vi "GUI_Sam_temp.vi"() -> ()   [LabVIEW 2013]
uses:
  shared programs/GUI_Template/GUI_master/tcp_new_data_event.ctl
  shared programs/GUI_Template/GUI_master/tcp new data cluster.ctl
panel:
  out "image::7":T1(plugin-control) caption="U_Amp3GaiaBay"
  in  "triggerdelay::7":dbl=0.001 caption="triggerdelay" min=0.0 max=50000.0 format="%_4p"
  in  "triggerdelay::6":dbl=0.001 caption="triggerdelay" min=20.0 max=50000.0 format="%_4p"
  in  "triggerdelay::5":dbl=0.001 caption="triggerdelay" min=10.0 max=50000.0 format="%_4p"
  in  "triggerdelay::4":dbl=0.001 caption="triggerdelay" min=0.0 max=50000.0 format="%_4p"
  in  "triggerdelay::3":dbl=0.001 caption="triggerdelay" min=20.0 max=50000.0 format="%_4p"
  in  "triggerdelay::2":dbl=0.001 caption="triggerdelay" min=0.0 max=50000.0 format="%_4p"
  in  "trigger::7":bool caption="Trigger"
  in  "centroidy::7":dbl=0.001 caption="centroid y" min=0.0 max=0.0 format="%_4f"
  in  "centroidx::7":dbl=0.001 caption="centroid x" min=0.0 max=0.0 format="%_4f"
  in  "exposure::7":dbl=0.001 caption="exposure" min=0.0001 max=1.0 format="%_4p"
  in  "GUIdevice 7":string="U_GAIACam"
  in  "trigger::6":bool caption="Trigger"
  in  "centroidy::6":dbl=0.001 caption="centroid y" min=0.0 max=0.0 format="%_4f"
  in  "centroidx::6":dbl=0.001 caption="centroid x" min=0.0 max=0.0 format="%_4f"
  in  "exposure::6":dbl=0.001 caption="exposure" min=0.0001 max=1.0 format="%_4p"
  out "image::6":T1(plugin-control) caption="U_Amp3GaiaBay"
  in  "GUIdevice 6":string="U_Amp3GaiaBay"
  in  "trigger::5":bool caption="Trigger"
  in  "centroidy::5":dbl=0.001 caption="centroid y" min=0.0 max=0.0 format="%_4f"
  in  "centroidx::5":dbl=0.001 caption="centroid x" min=0.0 max=0.0 format="%_4f"
  in  "exposure::5":dbl=0.001 caption="exposure" min=0.0001 max=1.0 format="%_4p"
  out "image::5":T1(plugin-control) caption="U_Amp2GaiaBay"
  in  "GUIdevice 5":string="U_Amp2GaiaBay"
  in  "trigger::4":bool caption="Trigger"
  in  "centroidy::4":dbl=0.001 caption="centroid y" min=0.0 max=0.0 format="%_4f"
  in  "centroidx::4":dbl=0.001 caption="centroid x" min=0.0 max=0.0 format="%_4f"
  in  "exposure::4":dbl=0.001 caption="exposure" min=1e-06 max=1.0 format="%_4p"
  out "image::4":T1(plugin-control) caption="U_IRMobileImager"
  in  "GUIdevice 4":string="U_IRMobileImager"
  in  "trigger::3":bool caption="Trigger"
  in  "centroidy::3":dbl=0.001 caption="centroid y" min=0.0 max=0.0 format="%_4f"
  in  "centroidx::3":dbl=0.001 caption="centroid x" min=0.0 max=0.0 format="%_4f"
  in  "exposure::3":dbl=0.001 caption="exposure" min=0.0001 max=1.0 format="%_4p"
  out "image::3":T1(plugin-control) caption="Amp3_IR_Input"
  in  "GUIdevice 3":string="U_Amp3_IR_Input"
  in  "trigger::2":bool caption="Trigger"
  in  "centroidy::2":dbl=0.001 caption="centroid y" min=0.0 max=0.0 format="%_4f"
  in  "centroidx::2":dbl=0.001 caption="centroid x" min=0.0 max=0.0 format="%_4f"
  in  "exposure::2":dbl=0.001 caption="exposure" min=0.0001 max=1.0 format="%_4p"
  out "image::2":T1(plugin-control) caption="Amp2_IR_input"
  in  "GUIdevice 2":string="U_Amp2_IR_input"
  out "tcp data event":T2
  in  "Refresh Button":bool
  in  "Select device":string(combo)="FrogHPD"
  in  "stop":bool
  in  "GUIdevice 1":string="HPD_CCD"
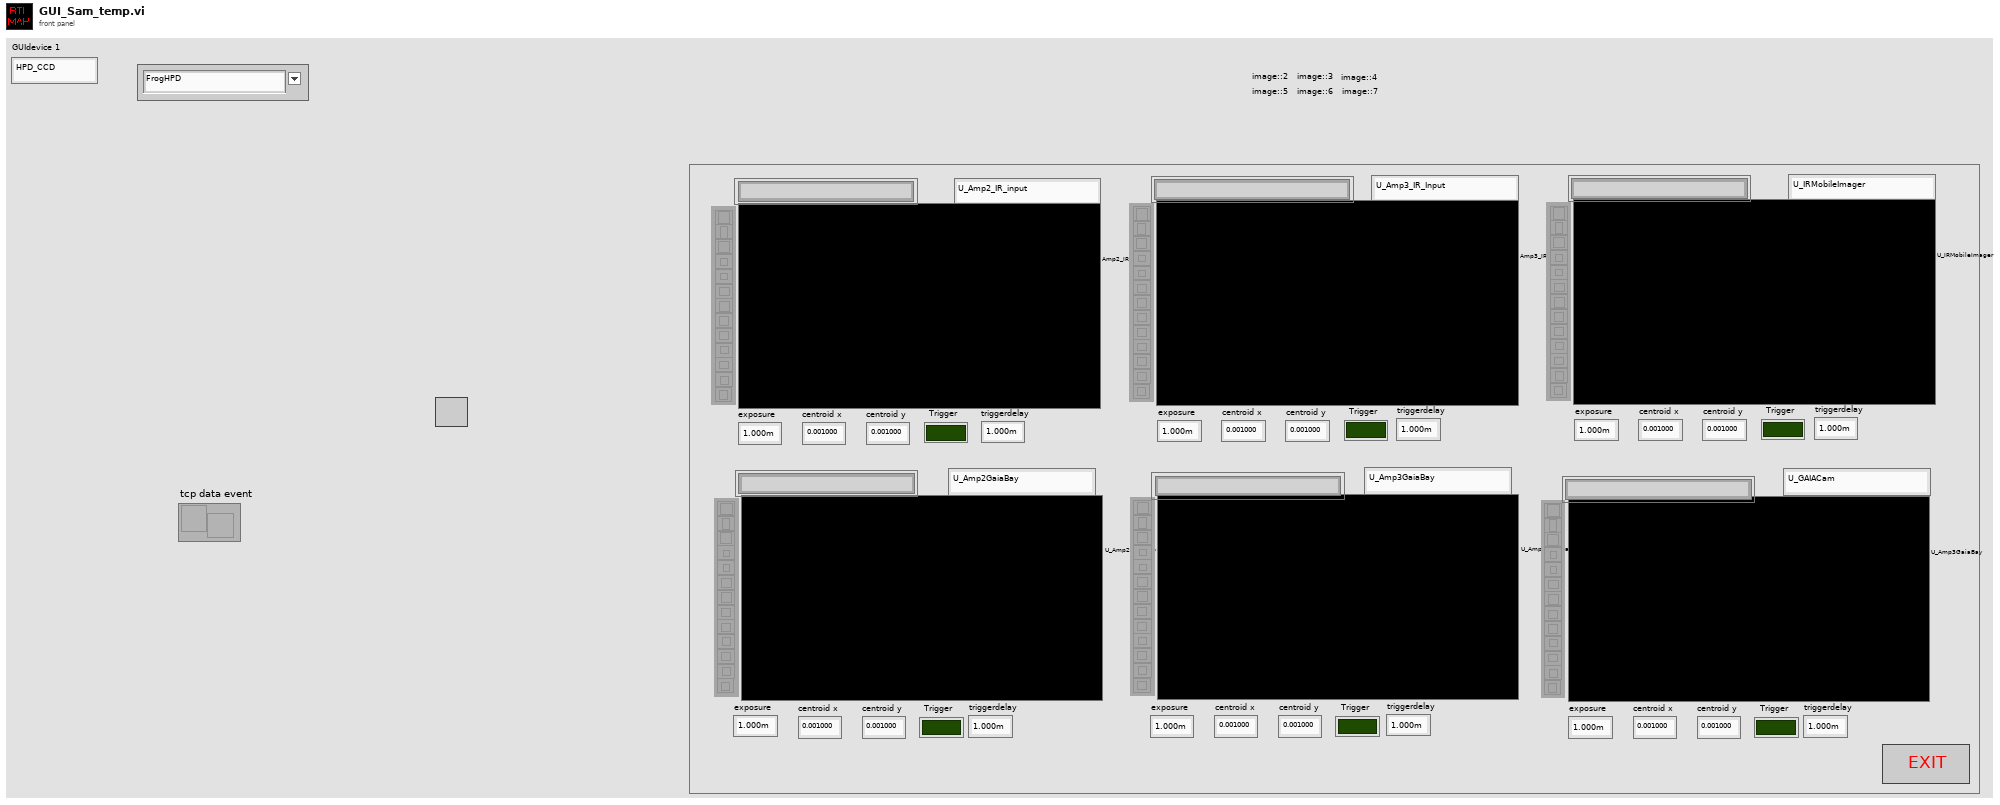
[diagram p1: front panel]
types:
  T1 = typedef "IMAQ Image.ctl" = refnum<image>
  T2 = typedef "tcp_new_data_event.ctl" = refnum<user-event>
  T3 = typedef "Image Type" = u32
  T4 = enum32{"invalid app kind", "Development System", "Run Time System", "Student Edition", "Embedded LabVIEW", "Evaluation", "Custom"}
  T5 = typedef "tcp new data cluster.ctl" = cluster{"EventEnum":enum16{"new data", "connection status update"}, "Device name":string}
  T6 = enum32{"Invalid", "Standard", "Closed", "Hidden", "Minimized", "Maximized"}
  T7 = cluster{"Core":cluster{"Current VI Reference":refnum<vi>, "Close Panel on Exit?":bool}, "Your Boolean data":bool, "Your string data":string, "SuperGUI":cluster{"STOP queue":refnum<queue>, "SuperGUI ref":refnum<vi>}}
  T8 = cluster{"STOP queue":refnum<queue>, "SuperGUI ref":refnum<vi>}
  T9 = cluster{"Current VI Reference":refnum<vi>, "Close Panel on Exit?":bool}
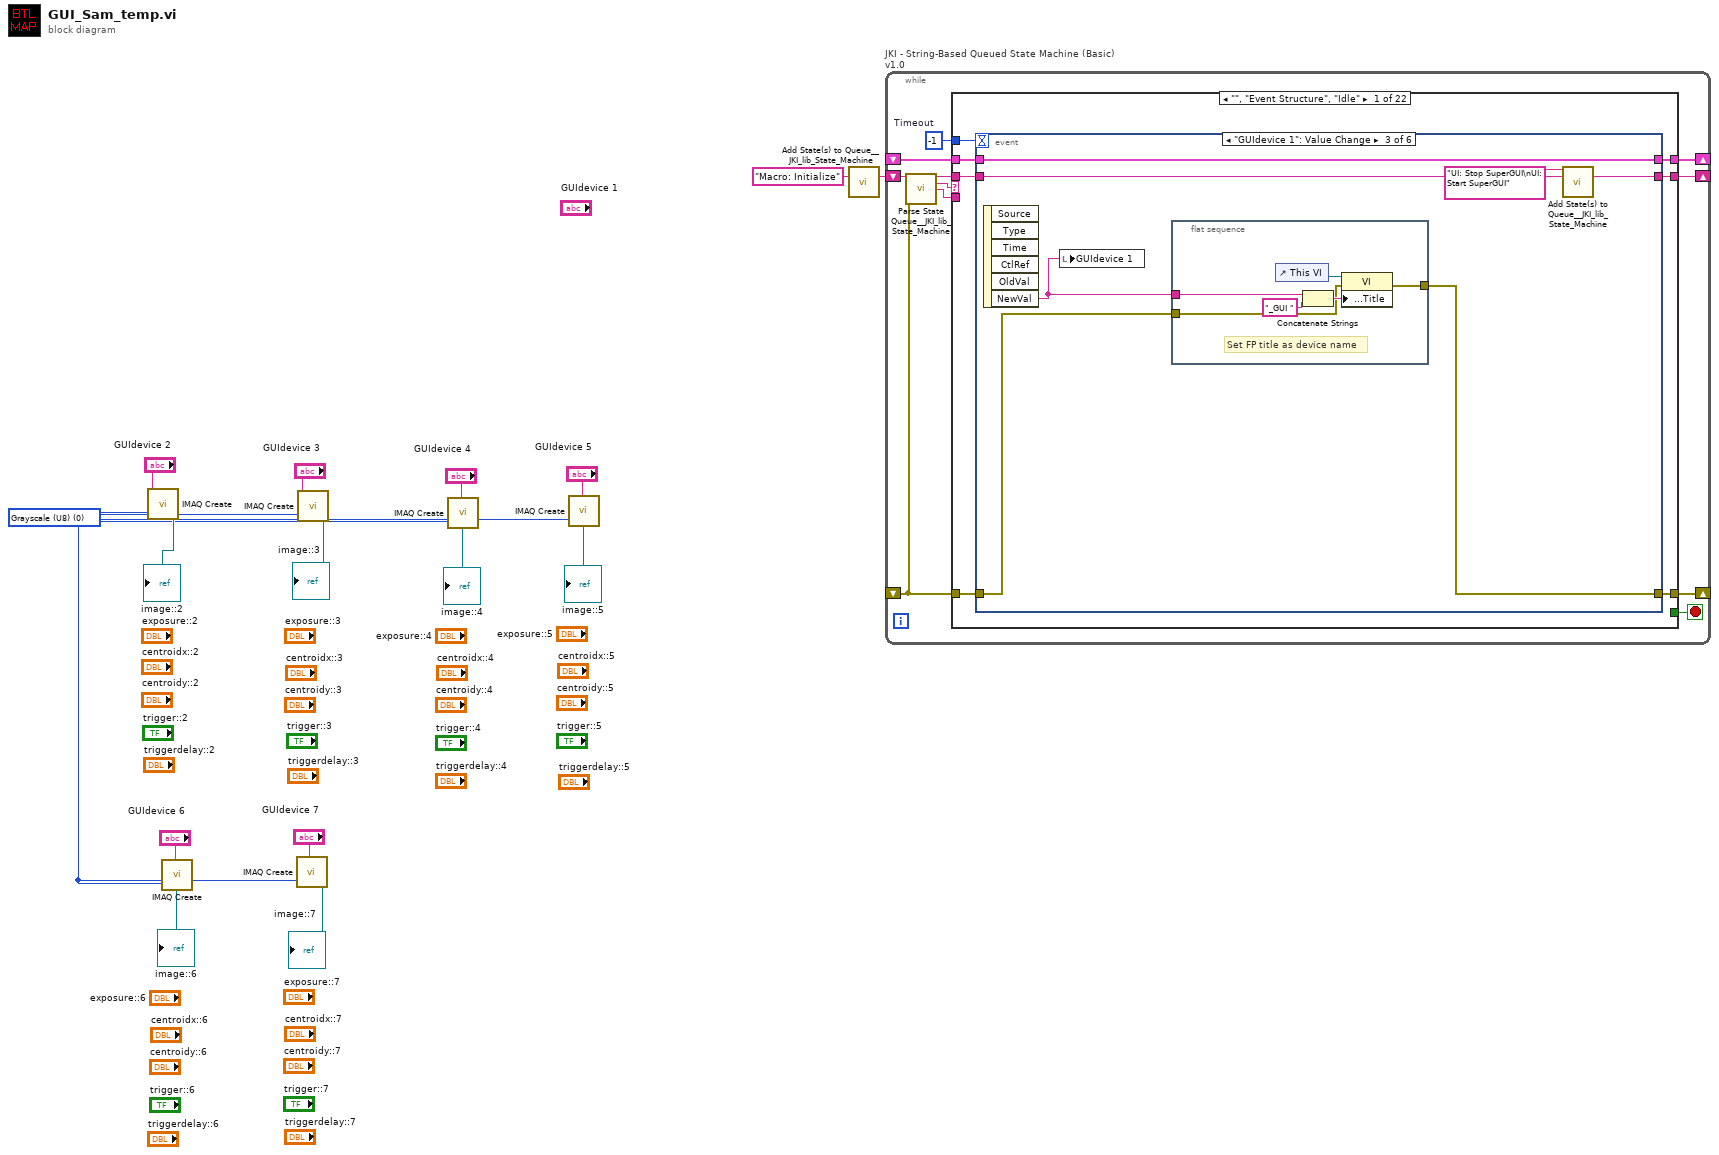
[diagram p0: block diagram]
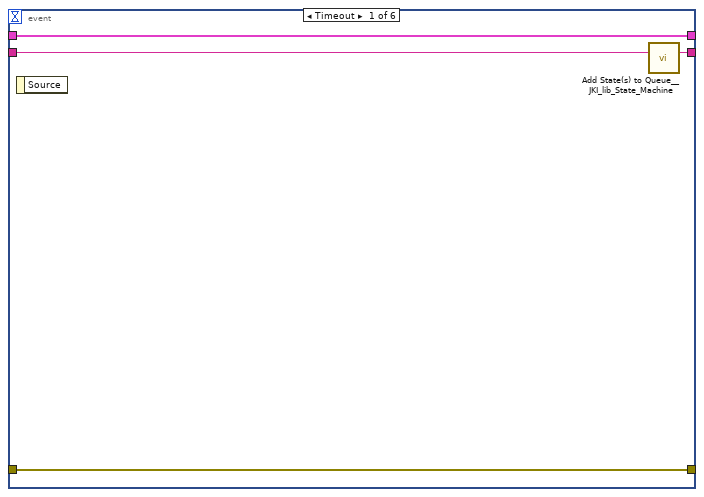
[diagram p2: hidden frame]
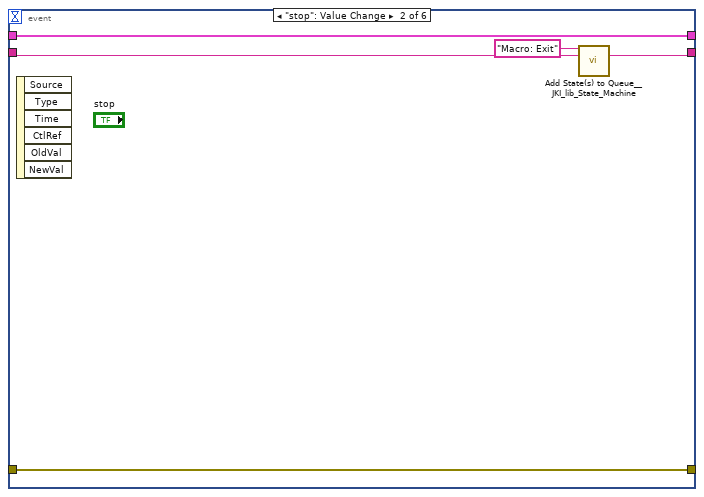
[diagram p3: hidden frame]
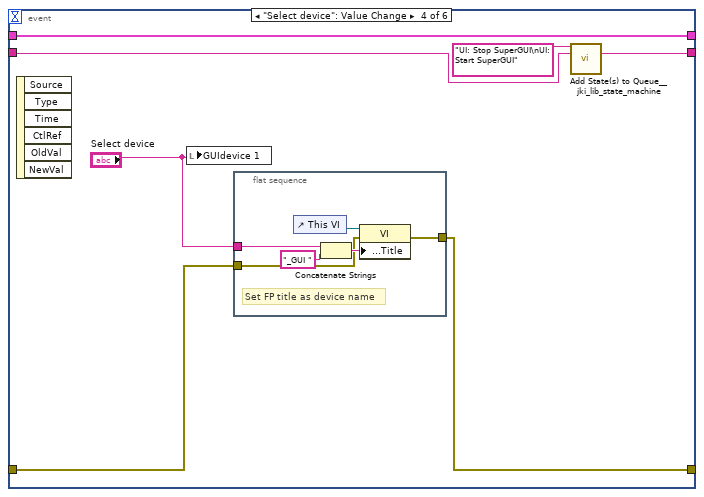
[diagram p4: hidden frame]
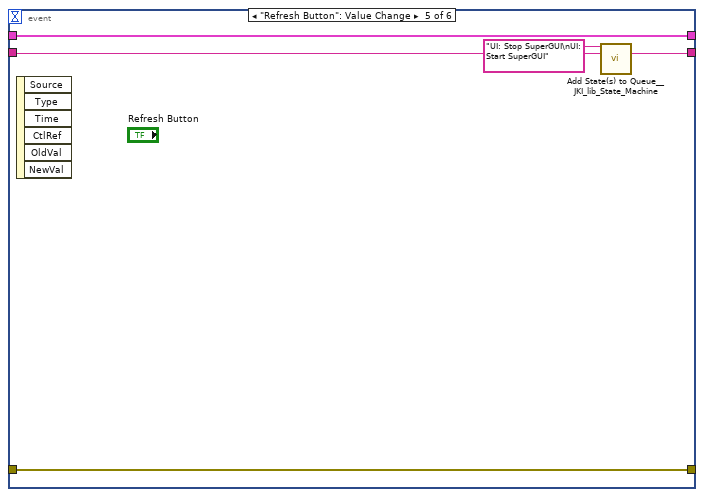
[diagram p5: hidden frame]
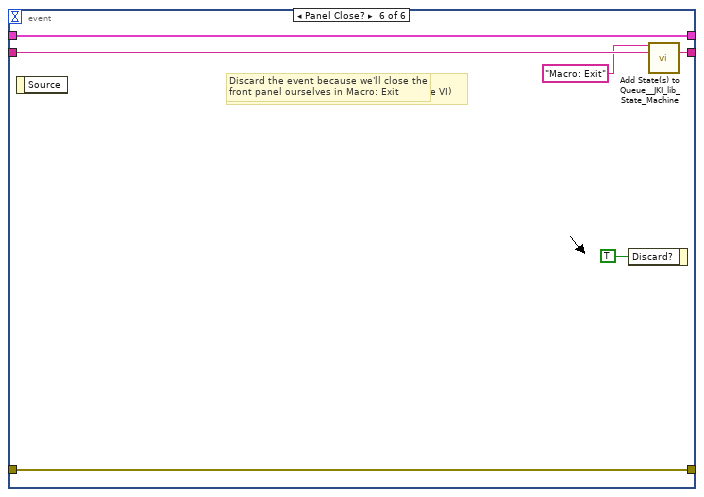
[diagram p6: hidden frame]
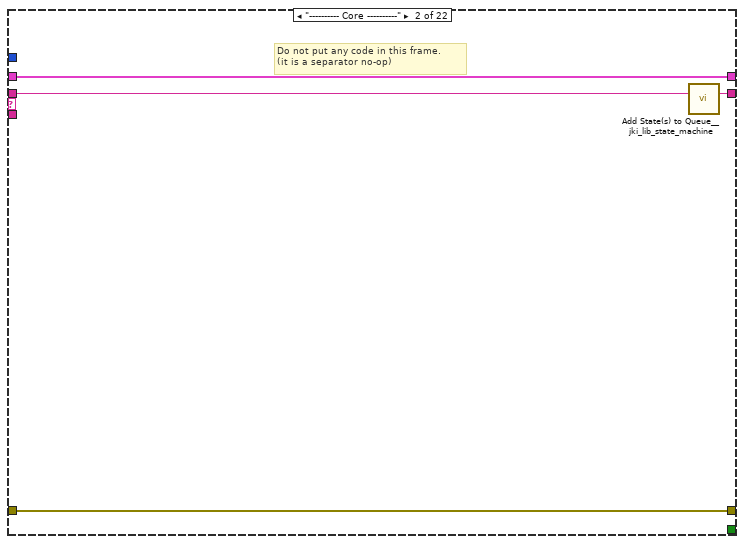
[diagram p7: hidden frame]
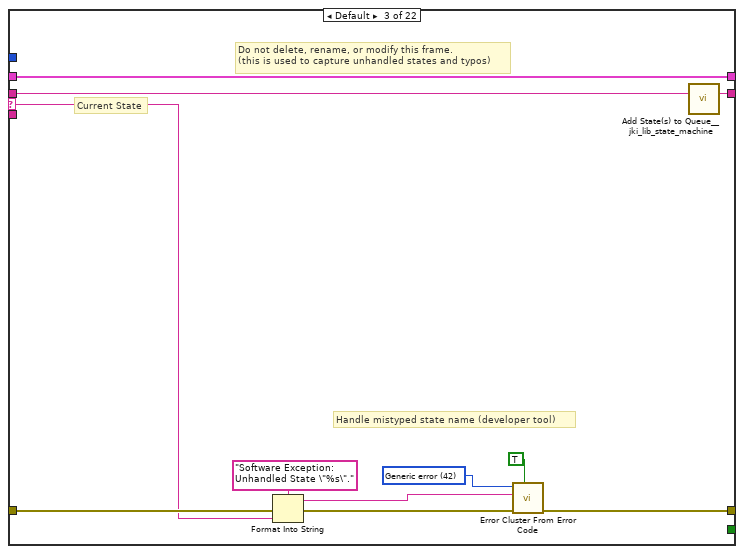
[diagram p8: hidden frame]
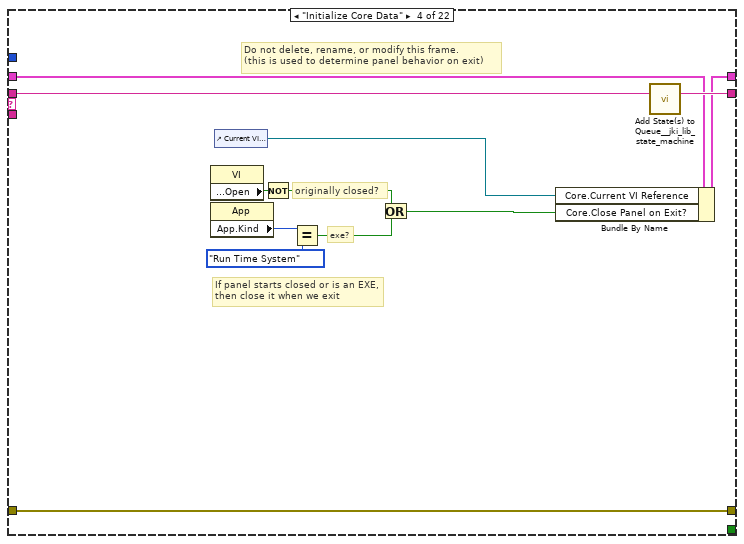
[diagram p9: hidden frame]
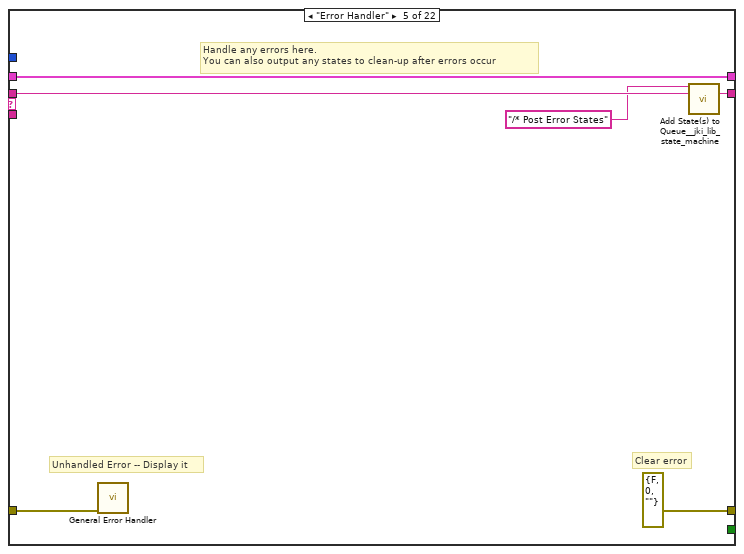
[diagram p10: hidden frame]
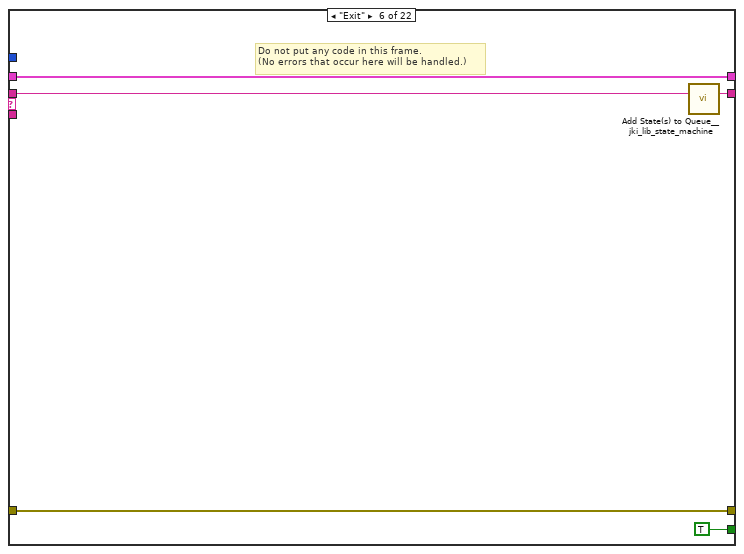
[diagram p11: hidden frame]
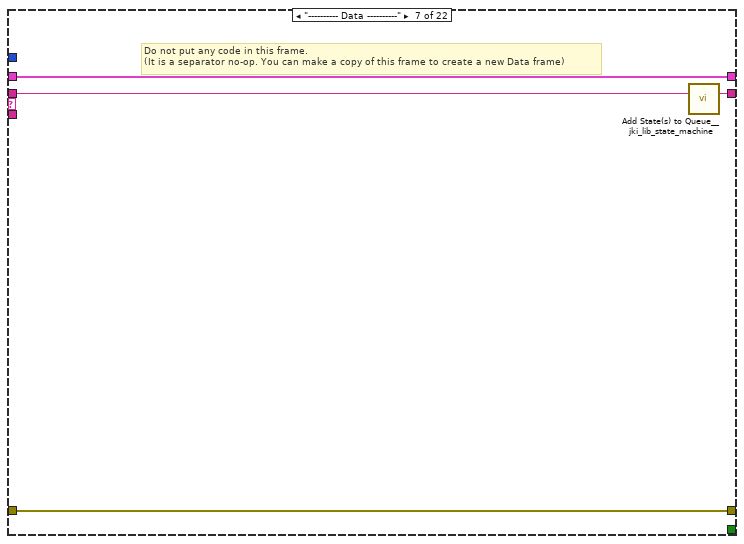
[diagram p12: hidden frame]
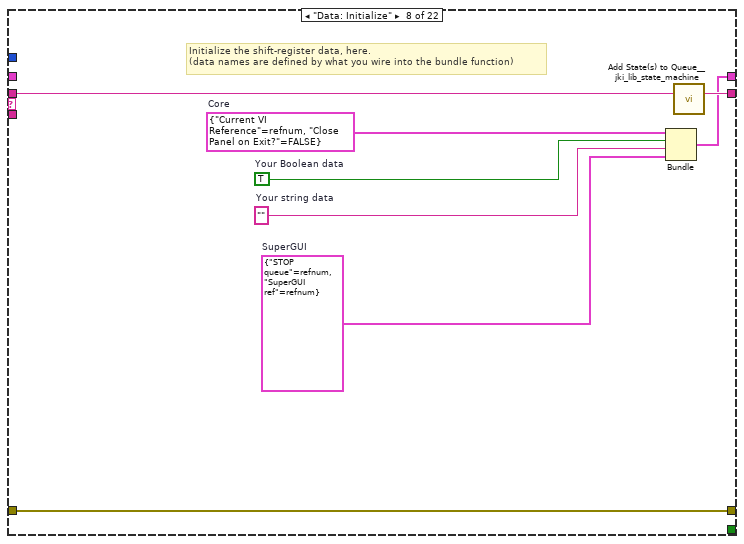
[diagram p13: hidden frame]
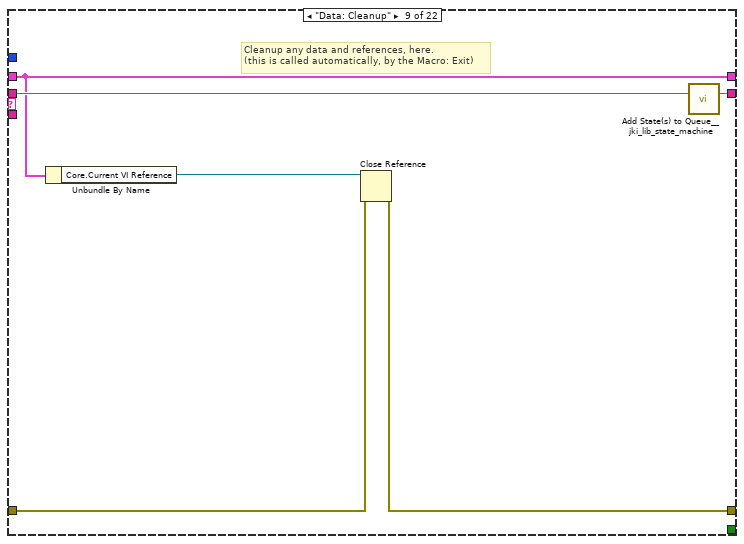
[diagram p14: hidden frame]
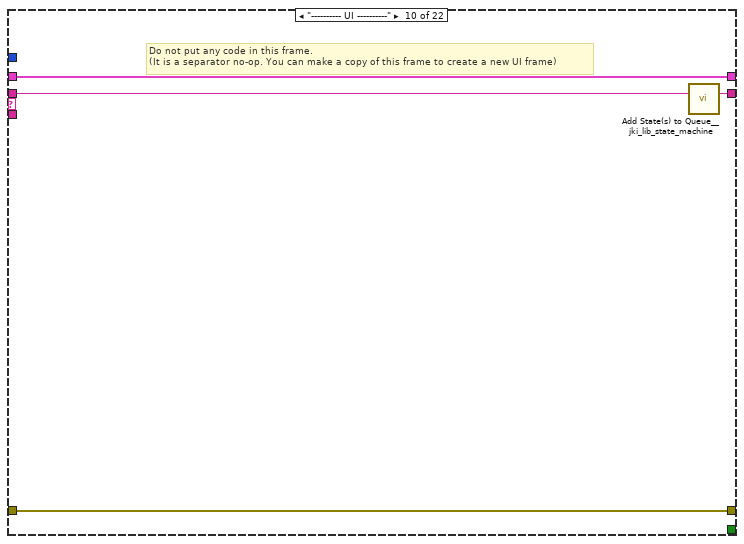
[diagram p15: hidden frame]
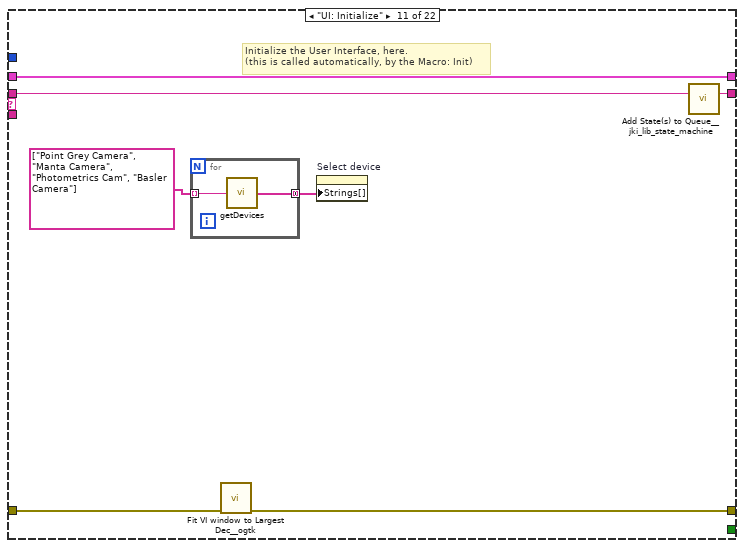
[diagram p16: hidden frame]
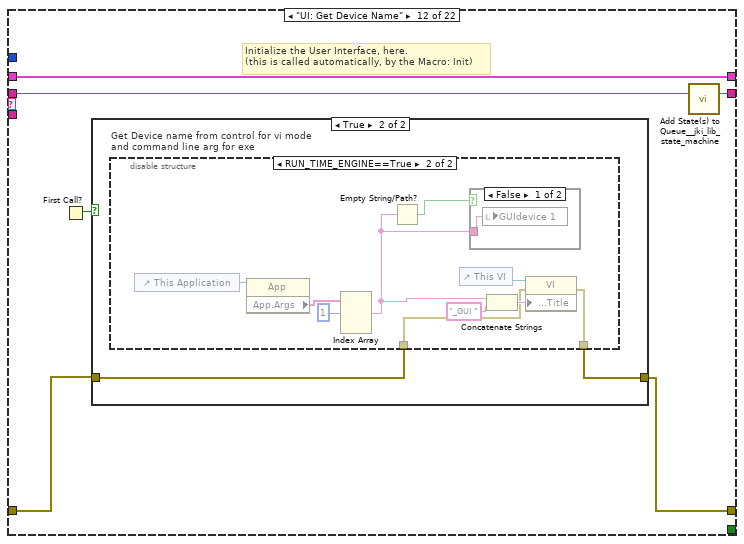
[diagram p17: hidden frame]
diagram:
  w2 = T3 0 items=["Grayscale (U8)", "Grayscale (I16)", "Grayscale (SGL)", "Complex (CSG)", "RGB (U32)", "HSL (U32)", "RGB (U64)", "Grayscale (U16)"] ("Image Type")
  n1 = call "IMAQ Create"("Image Name"="GUIdevice 2", "Image Type"=w2) -> ("New Image"=→"image::2":T1)  [unwired: 3 in, 1 out]
  n2 = call "IMAQ Create"("Image Name"="GUIdevice 6", "Image Type"=w2) -> ("New Image"=→"image::6":T1)  [unwired: 3 in, 1 out]
  n3 = call "IMAQ Create"("Image Name"="GUIdevice 7", "Image Type"=w2) -> ("New Image"=→"image::7":T1)  [unwired: 3 in, 1 out]
  n4 = call "IMAQ Create"("Image Name"="GUIdevice 3", "Image Type"=w2) -> ("New Image"=→"image::3":T1)  [unwired: 3 in, 1 out]
  n5 = call "IMAQ Create"("Image Name"="GUIdevice 4", "Image Type"=w2) -> ("New Image"=→"image::4":T1)  [unwired: 3 in, 1 out]
  n6 = call "IMAQ Create"("Image Name"="GUIdevice 5", "Image Type"=w2) -> ("New Image"=→"image::5":T1)  [unwired: 3 in, 1 out]
  n7 = call <vilib>:"Add State(s) to Queue__JKI_lib_State_Machine.vi"("State(s) in (\"\")"="Macro: Initialize") -> ("States Out"=w15:string)  [unwired: 14 in]
  n8 = while "JKI - String-Based Queued State Machine (Basic) v1.0" {
    shift-right: [w19] -> _
    shift-left: _ -> [w18]
    shift-right: [w22] -> _
    shift-left: _ -> [w16]
    shift-right: [w21] -> _
    shift-left: w15 -> [w23]
    stop <- w20 stop-if-true
    w17 = -1  # Timeout
    n9 = call <vilib>:"Parse State Queue__JKI_lib_State_Machine.vi"("State Queue"=w23, "Error In (no error)"=w16) -> ("Remaining States"=w25:string, "Current State"=w26:string, "Arguments"=w24:string)  [unwired: 11 in]
    n10 = case shown="\"\", \"Event Structure\", \"Idle\"" w26 {
      selector: w26 -> [_ _ w84 _ _ _ _ _ _ _ _ _ _ _ _ _ _ _ _ _ _ _]
      tunnel: w25 -> [w33 w83 w88 w106 w112 w117 w121 w129 w135 w139 w146 w154 w189 w197 w203 w214 w240 w245 w255 w259 w263 w267]
      tunnel: w24 -> [_ _ _ _ _ _ _ _ _ _ _ _ _ _ w198 w208 _ _ _ _ _ _]
      tunnel: w18 -> [w31 w80 w86 w97 w109 w115 w118 _ w130 w136 w144 w152 w180 w192 w201 w210 w237 w242 w252 w256 w260 w264]
      tunnel: [w30 w81 w90 w103 errorcluster {"status"=FALSE, "code"=0, "source"=""} ("error out") w114 w119 w126 w131 w137 w142 w149 w173 w190 w199 w211 w238 w243 w253 w257 w261 w265] -> w22
      tunnel: w16 -> [w29 w81 w89 w103 w108 w114 w119 w126 w132 w137 w143 w150 w174 w191 w200 w212 w238 w243 w253 w257 w261 w265]
      tunnel: [w32 w82 w87 w105 w111 w116 w120 w128 w134 w138 w145 w153 w188 w196 w202 w213 w239 w244 w254 w258 w262 w266] -> w21
      tunnel: [_ _ _ _ _ TRUE _ _ _ _ _ _ _ _ _ _ _ _ _ _ _ _] -> w20
      tunnel: [w28 w80 w86 w104 w109 w115 w118 w127 w130 w136 w144 w152 w179 w192 w201 w210 w237 w242 w252 w256 w260 w264] -> w19
      tunnel: w17 -> [w27 _ _ _ _ _ _ _ _ _ _ _ _ _ _ _ _ _ _ _ _ _]
      frame "", "Event Structure", "Idle" {
        n11 = event shown="[2] \"GUIdevice 1\": Value Change" {
          selector: _ -> [_ _ _ _ _ _]
          dyn-events: _ -> [_ _ _ _ _ _]
          timeout: w27 -> [_ _ _ _ _ _]
          tunnel: w33 -> [w37 w40 w46 w58 w71 w79]
          tunnel: [w36 w39 w45 w57 w70 w78] -> w32
          tunnel: w31 -> [w34 w42 w49 w62 w73 w76]
          tunnel: [w35 w41 w47 w60 w72 w77] -> w30
          tunnel: w29 -> [w35 w41 w48 w61 w72 w77]
          tunnel: [w34 w42 w49 w62 w73 w76] -> w28
          event Timeout {
            n12 = event-data() -> ()  [unwired: 1 in, 1 out]
            n13 = call <vilib>:"Add State(s) to Queue__JKI_lib_State_Machine.vi"("State(s) in (\"\")"=w37) -> ("States Out"=w36:string)  [unwired: 14 in]
          }
          event "stop": Value Change {
            n14 = event-data() -> ()  [unwired: 1 in, 6 out]
            n15 = call <vilib>:"Add State(s) to Queue__JKI_lib_State_Machine.vi"("State(s) in Front (\"\")"="Macro: Exit", "State(s) in (\"\")"=w40) -> ("States Out"=w39:string)  [unwired: 13 in]
          }
          event "GUIdevice 1": Value Change {
            n16 = event-data() -> ("NewVal"=w43:string)  [unwired: 1 in, 5 out]
            n17 = local write "GUIdevice 1"(w43) -> ()
            n18 = flat-sequence {
              tunnel: [w52] -> w47
              tunnel: w48 -> [w51]
              tunnel: w43 -> [w50]
              frame #0 {
                # "Set FP title as device name"
                n19 = control-ref of="This VI"() -> (w55:refnum<vi>)
                n20 = Concatenate Strings(w50, "_GUI ") -> (w54:string)
                n21 = property class="VI"(reference=w55, error in=w51, "Front Panel.Title"=w54) -> (error out=w52:errorcluster)  [unwired: 1 out]
              }
            }
            n22 = call <vilib>:"Add State(s) to Queue__JKI_lib_State_Machine.vi"("State(s) in Front (\"\")"="UI: Stop SuperGUI\nUI: Start SuperGUI", "State(s) in (\"\")"=w46) -> ("States Out"=w45:string)  [unwired: 13 in]
          }
          event "Select device": Value Change {
            n23 = event-data() -> ()  [unwired: 1 in, 6 out]
            n24 = local write "GUIdevice 1"("Select device") -> ()
            n25 = flat-sequence {
              tunnel: [w65] -> w60
              tunnel: w61 -> [w64]
              tunnel: "Select device" -> [w63]
              frame #0 {
                # "Set FP title as device name"
                n26 = control-ref of="This VI"() -> (w68:refnum<vi>)
                n27 = Concatenate Strings(w63, "_GUI ") -> (w67:string)
                n28 = property class="VI"(reference=w68, error in=w64, "Front Panel.Title"=w67) -> (error out=w65:errorcluster)  [unwired: 1 out]
              }
            }
            n29 = call <vilib>:"Add State(s) to Queue__jki_lib_state_machine.vi"("State(s) in Front (\"\")"="UI: Stop SuperGUI\nUI: Start SuperGUI", "State(s) in (\"\")"=w58) -> ("States Out"=w57:string)  [unwired: 13 in]
          }
          event "Refresh Button": Value Change {
            n30 = event-data() -> ()  [unwired: 1 in, 6 out]
            n31 = call <vilib>:"Add State(s) to Queue__JKI_lib_State_Machine.vi"("State(s) in Front (\"\")"="UI: Stop SuperGUI\nUI: Start SuperGUI", "State(s) in (\"\")"=w71) -> ("States Out"=w70:string)  [unwired: 13 in]
          }
          event Panel Close? {
            # "Discard the event because we'll close the front panel ourselves in Macro: Exit"
            # "Close Panel button (pressed) Event\n(this executes Macro: Exit to terminate the VI)"
            n32 = event-data() -> ()  [unwired: 1 in, 1 out]
            n33 = event-data("Discard?"=TRUE) -> ()  [unwired: 1 in, 1 out]
            n34 = call <vilib>:"Add State(s) to Queue__JKI_lib_State_Machine.vi"("State(s) in Front (\"\")"="Macro: Exit", "State(s) in (\"\")"=w79) -> ("States Out"=w78:string)  [unwired: 13 in]
          }
        }
      }
      frame "---------- Core ----------" {
        # "Do not put any code in this frame.\n(it is a separator no-op)"
        n35 = call <vilib>:"Add State(s) to Queue__jki_lib_state_machine.vi"("State(s) in (\"\")"=w83) -> ("States Out"=w82:string)  [unwired: 14 in]
      }
      frame Default {
        w93 = 42 items=["No error", "Argument error", "Memory is full", "Out of zone", "End of file", "File already open", "Generic file I/O error", "File not found", "File permission error", "Disk is full", "Duplicate path", "Too many files open", "System feature not enabled", "Resource file not found", "Cannot add resource", "Resource not found", "Image not found", "Image memory error", "Pen does not exist", "Config type invalid", "Config token not found", "Config parse error", "Config memory error", "Bad external code format", "Bad external code offset", "External code not present", "Null window", "Destroy window error", "Null menu", "Print aborted", "Bad print record", "Print driver error", "Windows error during printing", "Memory error during printing", "Print dialog error", "Generic print error", "Invalid device refnum", "Device not found", "Device parameter error", "Device unit error", "Cannot open device", "Device call aborted", "Generic error", "Cancelled by user", "Object ID too low", "Object ID too high", "Object not in heap", "Unknown heap", "Unknown object (invalid DefProc)", "Unknown object (DefProc not in table)", "Message out of range", "Invalid (null) method", "Unknown message", "Manager call not supported", "Bad address", "Network operation in progress", "Network operation timed out", "Connection is busy", "Network attribute not supported", "Network error", "Address in use", "System out of memory", "Connection aborted", "Connection refused", "Not connected", "Already connected", "Connection closed", "Initialization error (interapplication manager)", "Bad occurrence", "Wait on unbound occurrence handler", "Occurrence queue overflow", "Datalog type conflict", "Unused", "Unrecognized type (interapplication manager)", "Memory corrupt", "Failed to make temporary DLL", "Old CIN version", "Drag socket not found", "Failed to load drop-object", "Failed to register OLE object", "Failed to release OLE object", "Format specifier type mismatch", "Unknown format specifier", "Too few format specifiers", "Too many format specifiers", "Scan failed", "Newer CIN version", "Error converting to variant", "Runtime menu error", "Password tampered", "Variant attribute not found", "Incompatible variant data type", "Event data is not available", "Event Store is not present", "Occurrence is not found", "Event Queue is not created", "Event info is not available", "Refnum passed is NULL", "Error retrieving Class GUID", "Error retrieving CoClass GUID", "Error retrieving TypeLib GUID.", "Bad built application magic bytes.", "Specific driver is different from the specific driver associated with the Logical Name.", "There is no session opened to the class driver.", "Max Error", "MAX - Error with config objects", "MAX - Error loading configuration", "MAX - Group not supported"]
        # "Current State"
        # "Do not delete, rename, or modify this frame.\n(this is used to capture unhandled states and typos)"
        # "Handle mistyped state name (developer tool)"
        n36 = Format Into String(format string="Software Exception: Unhandled State \"%s\"." ("message"), error in=w89, w84) -> (resulting string=w92:string, error out=w91:errorcluster)  [unwired: 1 in]
        n37 = call <vilib>:"Error Cluster From Error Code.vi"("show call chain? (False)"=TRUE, "error in (no error)"=w91, "error message (\"\")"=w92, "error code (0)"=w93) -> ("error out"=w90:errorcluster)  [unwired: 5 in]
        n38 = call <vilib>:"Add State(s) to Queue__jki_lib_state_machine.vi"("State(s) in (\"\")"=w88) -> ("States Out"=w87:string)  [unwired: 14 in]
      }
      frame "Initialize Core Data" {
        # "Do not delete, rename, or modify this frame.\n(this is used to determine panel behavior on exit)"
        # "originally closed?"
        # "exe?"
        # "If panel starts closed or is an EXE, then close it when we exit"
        n39 = property class="VI"() -> ("Front Panel.Open"=w102:bool)  [unwired: 2 in, 2 out]
        n40 = property class="App"() -> ("App.Kind"=w101:T4)  [unwired: 2 in, 2 out]
        n41 = control-ref of="Current VI Reference"() -> (w95:refnum<vi>)
        n42 = Not(x=w102) -> (.not. x?=w99:bool)
        n43 = Equal?(x=w101, y=T4."Run Time System" ("Application:Kind")) -> (x = y?=w98:bool)
        n44 = Or(x=w99, y=w98) -> (x .or. y?=w96:bool)
        n45 = Bundle By Name(cluster=w97, "Core.Current VI Reference"=w95, "Core.Close Panel on Exit?"=w96) -> (w104:T7)
        n46 = call <vilib>:"Add State(s) to Queue__jki_lib_state_machine.vi"("State(s) in (\"\")"=w106) -> ("States Out"=w105:string)  [unwired: 14 in]
      }
      frame "Error Handler" {
        # "Unhandled Error -- Display it"
        # "Handle any errors here.\nYou can also output any states to clean-up after errors occur"
        # "Clear error"
        n47 = call <vilib>:"General Error Handler.vi"("error in (no error)"=w108) -> ()  [unwired: 10 in, 5 out]
        n48 = call <vilib>:"Add State(s) to Queue__jki_lib_state_machine.vi"("State(s) in Front (\"\")"="/* Post Error States", "State(s) in (\"\")"=w112) -> ("States Out"=w111:string)  [unwired: 13 in]
      }
      frame "Exit" {
        # "Do not put any code in this frame.\n(No errors that occur here will be handled.)"
        n49 = call <vilib>:"Add State(s) to Queue__jki_lib_state_machine.vi"("State(s) in (\"\")"=w117) -> ("States Out"=w116:string)  [unwired: 14 in]
      }
      frame "---------- Data ----------" {
        # "Do not put any code in this frame.\n(It is a separator no-op. You can make a copy of this frame to create a new Data frame)"
        n50 = call <vilib>:"Add State(s) to Queue__jki_lib_state_machine.vi"("State(s) in (\"\")"=w121) -> ("States Out"=w120:string)  [unwired: 14 in]
      }
      frame "Data: Initialize" {
        w122 = T8 {"STOP queue"=refnum, "SuperGUI ref"=refnum}  # SuperGUI
        w123 = T9 {"Current VI Reference"=refnum, "Close Panel on Exit?"=FALSE}  # Core
        w125 = TRUE  # Your Boolean data
        w124 = ""  # Your string data
        # "Initialize the shift-register data, here.\n(data names are defined by what you wire into the bundle function)"
        n51 = Bundle("Core"=w123, "Your Boolean data"=w125, "Your string data"=w124, "SuperGUI"=w122) -> (w127:T7)  [unwired: 1 in]
        n52 = call <vilib>:"Add State(s) to Queue__jki_lib_state_machine.vi"("State(s) in (\"\")"=w129) -> ("States Out"=w128:string)  [unwired: 14 in]
      }
      frame "Data: Cleanup" {
        # "Cleanup any data and references, here.\n(this is called automatically, by the Macro: Exit)"
        n53 = Unbundle By Name(w130) -> ("Core.Current VI Reference"=w133:refnum<vi>)
        n54 = Close Reference(reference=w133, error in (no error)=w132) -> (error out=w131:errorcluster)
        n55 = call <vilib>:"Add State(s) to Queue__jki_lib_state_machine.vi"("State(s) in (\"\")"=w135) -> ("States Out"=w134:string)  [unwired: 14 in]
      }
      frame "---------- UI ----------" {
        # "Do not put any code in this frame.\n(It is a separator no-op. You can make a copy of this frame to create a new UI frame)"
        n56 = call <vilib>:"Add State(s) to Queue__jki_lib_state_machine.vi"("State(s) in (\"\")"=w139) -> ("States Out"=w138:string)  [unwired: 14 in]
      }
      frame "UI: Initialize" {
        # "Initialize the User Interface, here.\n(this is called automatically, by the Macro: Init)"
        n57 = for {
          tunnel: string[] ["Point Grey Camera", "Manta Camera", "Photometrics Cam", "Basler Camera"] -> [w148] mode=indexing
          tunnel: [w147] -> w140 mode=concatenating
          n58 = call "getDevices.vi"("Device Class"=w148) -> ("All Devices"=w147:string[])
        }
        n59 = call <userlib>:"Fit VI window to Largest Dec__ogtk.vi"("error in (no error)"=w143) -> ("error out"=w142:errorcluster)  [unwired: 5 in, 1 out]
        n60 = property on="Select device" class="CmbBox"("Strings[]"=w140) -> ()  [unwired: 2 in, 2 out]
        n61 = call <vilib>:"Add State(s) to Queue__jki_lib_state_machine.vi"("State(s) in (\"\")"=w146) -> ("States Out"=w145:string)  [unwired: 14 in]
      }
      frame "UI: Get Device Name" {
        # "Initialize the User Interface, here.\n(this is called automatically, by the Macro: Init)"
        n62 = First Call?() -> (First Call?: T/F=w151:bool)
        n63 = case shown="True" w151 {
          tunnel: w150 -> [w155 w157]
          tunnel: [w155 w156] -> w149
          frame False {
          }
          frame True {
            n64 = disable-structure "Get Device name from control for vi mode\nand command line arg for exe" shown="RUN_TIME_ENGINE==True" {
              disable-tunnel: w157 -> [w158 w160]
              disable-tunnel: [w158 w159] -> w156
              frame condition #0 (active) {
              }
              frame condition #1 {
                n65 = control-ref of="This Application"() -> (w168:refnum<vi>)
                n66 = property class="App"(reference=w168) -> ("App.Args"=w167:string[])  [unwired: 1 in, 2 out]
                n67 = Index Array(array=w167, index #1=1 ("index")) -> (element #1=w161:string)  [unwired: 2 in, 2 out]
                n68 = Empty String/Path?(string/path=w161) -> (empty?=w165:bool)
                n69 = control-ref of="This VI"() -> (w164:refnum<vi>)
                n70 = case shown="False" w165 {
                  tunnel: w161 -> [w169 _]
                  frame False {
                    n71 = local write "GUIdevice 1"(w169) -> ()
                  }
                  frame True {
                  }
                }
                n72 = Concatenate Strings(w161, "_GUI ") -> (w163:string)
                n73 = property class="VI"(reference=w164, error in=w160, "Front Panel.Title"=w163) -> (error out=w159:errorcluster)  [unwired: 1 out]
              }
            }
          }
        }
        n74 = call <vilib>:"Add State(s) to Queue__jki_lib_state_machine.vi"("State(s) in (\"\")"=w154) -> ("States Out"=w153:string)  [unwired: 14 in]
      }
      frame "UI: Start SuperGUI" {
        # "create stop queue for supergui and its clones"
        # "x100 abort will be dependent on caller VI\nx80 abort will be independent of caller vi, this will abort vi when labview is closed."
        # "Start SuperGUI asynchronous way"
        n75 = vi-ref "GUI_Master_subvi_reentrant_queues.vi"() -> (w172:refnum<vi>)
        n76 = property class="VI"(reference=w172) -> ("Path"=w171:path)  [unwired: 1 in, 2 out]
        n77 = Create User Event(user event datatype=T5 {"EventEnum"=enum."new data", "Device name"="Device name"} ("New Event"), error in=w174) -> (user event=w175:refnum<user-event>, error out=w181:errorcluster)
        "tcp data event" <- w175
        n78 = control-ref of="This Application"() -> (w178:refnum<vi>)
        n79 = control-ref of="This VI"() -> (w177:refnum<vi>)
        n80 = Open VI Reference(type specifier VI Refnum (for type only)=refnum<vi> refnum, vi path=w171, options=256) -> (vi reference=w187:refnum<vi>, error out=w186:errorcluster)  [unwired: 3 in]
        n81 = register-events(w175) -> ()  [unwired: 2 in, 2 out]
        n82 = call "supergui create stop queue.vi"() -> ("STOP Queue out"=w183:refnum<queue>)  [unwired: 11 in]
        n83 = Current VI's Menubar() -> (w176:refnum<k9>)
        n84 = call-by-ref "Start Asynchronous Call"(reference=w187, error in=w186, "STOP Queue in"=w183, "This Application"=w178, 8:"error in (no error)"=w181, "tcp data event"=w175, "Caller menu reference"=w176, "Caller VI ref"=w177) -> (reference out=w170:refnum<vi>, error out=w173:errorcluster)  [unwired: 5 in, 1 out]
        n85 = Bundle By Name(cluster=w180, "SuperGUI.SuperGUI ref"=w170, "SuperGUI.STOP queue"=w183) -> (w179:T7)
        n86 = call <vilib>:"Add State(s) to Queue__jki_lib_state_machine.vi"("State(s) in (\"\")"=w189) -> ("States Out"=w188:string)  [unwired: 14 in]
      }
      frame "UI: Stop SuperGUI" {
        # "Stop Supergui Clone and wait until it exit properly"
        n87 = Unbundle By Name(w192) -> ("SuperGUI.SuperGUI ref"=w194:refnum<vi>, "SuperGUI.STOP queue"=w193:refnum<queue>)
        n88 = Release Queue(queue=w193, error in (no error)=w191) -> (error out=w195:errorcluster)  [unwired: 1 in, 2 out]
        n89 = call-by-ref "Wait On Asynchronous Call"(reference=w194, error in=w195) -> ("error out"=w190:errorcluster)  [unwired: 11 in, 2 out]
        n90 = call <vilib>:"Add State(s) to Queue__jki_lib_state_machine.vi"("State(s) in (\"\")"=w197) -> ("States Out"=w196:string)  [unwired: 14 in]
      }
      frame "UI: Cursor Set" {
        # "Argument"
        # "Set and Unset Cursor Busy.\n(Usage: \"UI: Cursor Set >> Busy|Idle\")"
        n91 = case shown="\"Idle\", Default" w198 {
          tunnel: w200 -> [w205 w207]
          tunnel: [w204 w206] -> w199
          frame "Idle", Default {
            n92 = call <vilib>:"Unset Busy.vi"("error in (no error)"=w205) -> ("error out"=w204:errorcluster)  [unwired: 10 in]
          }
          frame "Busy" {
            n93 = call <vilib>:"Set Busy.vi"("error in (no error)"=w207) -> ("error out"=w206:errorcluster)  [unwired: 9 in, 1 out]
          }
        }
        n94 = call <vilib>:"Add State(s) to Queue__jki_lib_state_machine.vi"("State(s) in (\"\")"=w203) -> ("States Out"=w202:string)  [unwired: 14 in]
      }
      frame "UI: Front Panel State" {
        # "Argument"
        # "Set Front Panel Open or Closed\n(Usage: \"UI: Front Panel State >> Open|Close\")"
        n95 = Unbundle By Name(w210) -> ("Core.Current VI Reference"=w209:refnum<vi>)
        n96 = case shown="\"Open\", Default" w208 {
          tunnel: w212 -> [w218 w231]
          tunnel: [w220 w232] -> w211
          tunnel: w209 -> [w219 w229]
          frame "Open", Default {
            n97 = property class="VI"(reference=w219, error in=w218) -> (reference out=w216:refnum<vi>, error out=w217:errorcluster, "Front Panel.Open"=w215:bool)
            n98 = case shown="False" w215 {
              tunnel: [w223 w226] -> w220
              tunnel: w217 -> [w222 w226]
              tunnel: w216 -> [w221 _]
              frame False {
                n99 = invoke class="VI" method="FP.Open"(reference=w221, error in=w222, "Activate"=TRUE, "State"=T6."Standard") -> (error out=w223:errorcluster)  [unwired: 1 in, 4 out]
              }
              frame True {
              }
            }
          }
          frame "Close" {
            n100 = property class="VI"(reference=w229, error in=w231) -> (reference out=w228:refnum<vi>, error out=w230:errorcluster, "Front Panel.Open"=w227:bool)
            n101 = case shown="True" w227 {
              tunnel: [w233 w236] -> w232
              tunnel: w230 -> [w233 w235]
              tunnel: w228 -> [_ w234]
              frame False {
              }
              frame True {
                n102 = invoke class="VI" method="FP.Close"(reference=w234, error in=w235) -> (error out=w236:errorcluster)  [unwired: 1 in, 2 out]
              }
            }
          }
        }
        n103 = call <vilib>:"Add State(s) to Queue__jki_lib_state_machine.vi"("State(s) in (\"\")"=w214) -> ("States Out"=w213:string)  [unwired: 14 in]
      }
      frame "---------- Macro ----------" {
        # "Do not put any code in this frame.\n(It is a separator no-op. You can make a copy of this frame to create a new Macro frame)"
        n104 = call <vilib>:"Add State(s) to Queue__jki_lib_state_machine.vi"("State(s) in (\"\")"=w240) -> ("States Out"=w239:string)  [unwired: 14 in]
      }
      frame "Macro: Initialize" {
        # "Initialization Macro\n(This is called once, when the VI starts)"
        n105 = call <vilib>:"Add State(s) to Queue__jki_lib_state_machine.vi"("State(s) in Front (\"\")"="Data: Initialize\nInitialize Core Data\nUI: Initialize\nUI: Get Device Name\nUI: Start SuperGUI\nUI: Front Panel State >> Open", "State(s) in (\"\")"=w245) -> ("States Out"=w244:string)  [unwired: 13 in]
      }
      frame "Macro: Exit" {
        # "Exit Macro\n(This is called once, when the VI exits)"
        n106 = Unbundle By Name(w252) -> ("Core.Close Panel on Exit?"=w251:bool)
        n107 = Select(t="UI: Front Panel State >> Close", s=w251, f="") -> (s? t:f=w248:string)
        n108 = call <vilib>:"Add State(s) to Queue__jki_lib_state_machine.vi"("State(s) in (\"\")"=w248, "State(s) at Back (\"\")"="Data: Cleanup\nExit") -> ("States Out"=w246:string)  [unwired: 13 in]
        n109 = call <vilib>:"Add State(s) to Queue__jki_lib_state_machine.vi"("State(s) in Front (\"\")"=w246, "State(s) in (\"\")"=w255) -> ("States Out"=w254:string)  [unwired: 13 in]
      }
      frame "---------- New Category ----------" {
        # "Template Separator\n(You can make a copy of, or modify, this frame)"
        n110 = call <vilib>:"Add State(s) to Queue__jki_lib_state_machine.vi"("State(s) in (\"\")"=w259) -> ("States Out"=w258:string)  [unwired: 14 in]
      }
      frame "New Category: 1" {
        # "Your code here.\n(You can make a copy of, or modify, this frame)"
        n111 = call <vilib>:"Add State(s) to Queue__jki_lib_state_machine.vi"("State(s) in (\"\")"=w263) -> ("States Out"=w262:string)  [unwired: 14 in]
      }
      frame "New Category: 2" {
        # "Your code here.\n(You can make a copy of, or modify, this frame)"
        n112 = call <vilib>:"Add State(s) to Queue__jki_lib_state_machine.vi"("State(s) in (\"\")"=w267) -> ("States Out"=w266:string)  [unwired: 14 in]
      }
    }
  }
